vi "ITX to LV 2.2.vi"(0 "file (use dialog)":path=path "P:/sample/GaAs/GaAs quantum dots/2008/PL Map/A1 735/060731ASBA_A1_6.0.itx") -> (2 "2D array":dbl[][](array[numeric]), 3 "1D arrays":dbl[][](array[numeric]), 4 "wave names":string[](array[string]), 5 "Notes":string)   [LabVIEW 2016, in "LVtoITX.lvclass"]
uses:
  LVtoITX.lvclass
panel:
  out "variant to data (ms)":u32
  out "Commands":string
  out "parse 2 (ms)":u32
  out "text to data (ms)":u32
  out "parse 1 (ms)":u32
  out "open file (ms)":u32
  out "Array 4":i32[](array[numeric])
  out "Array":string[](array[string])
  out "array":string[](array[string])
  out "error out":errorcluster
  out "logical AND":bool
  out "Array 2":string[](array[string])
  out "spreadsheet strings":string[](array[string])
  in  "error in":errorcluster
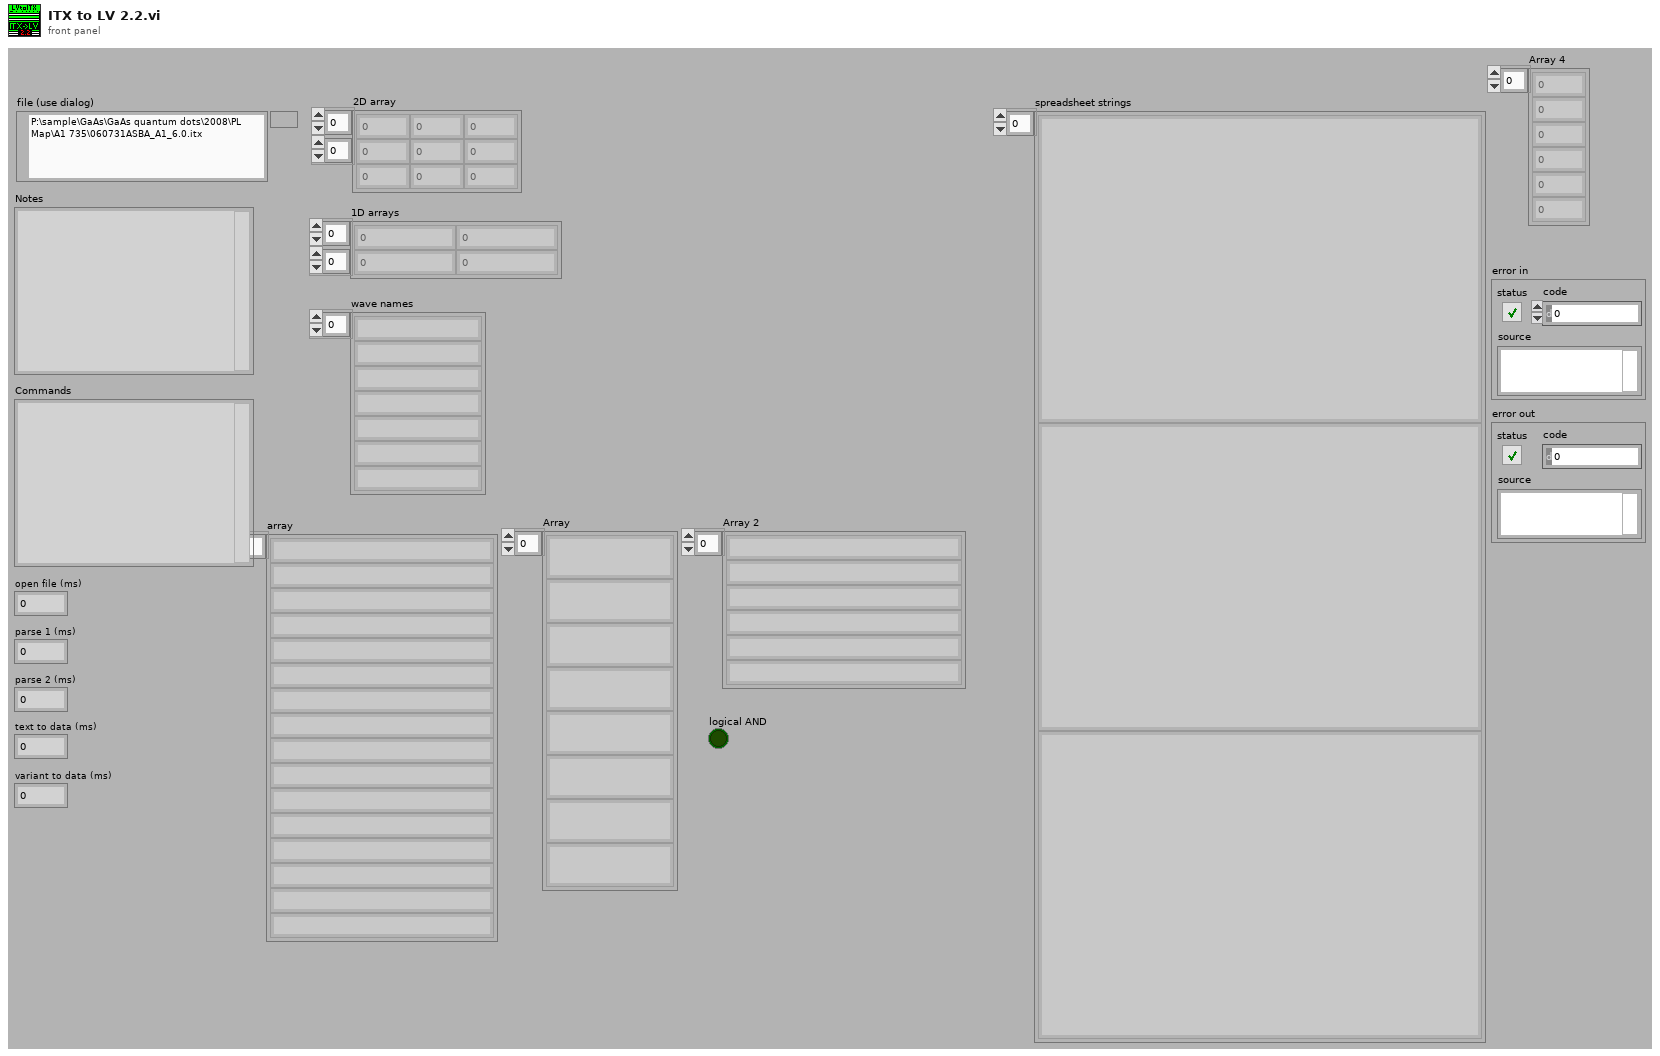
[diagram p1: front panel]
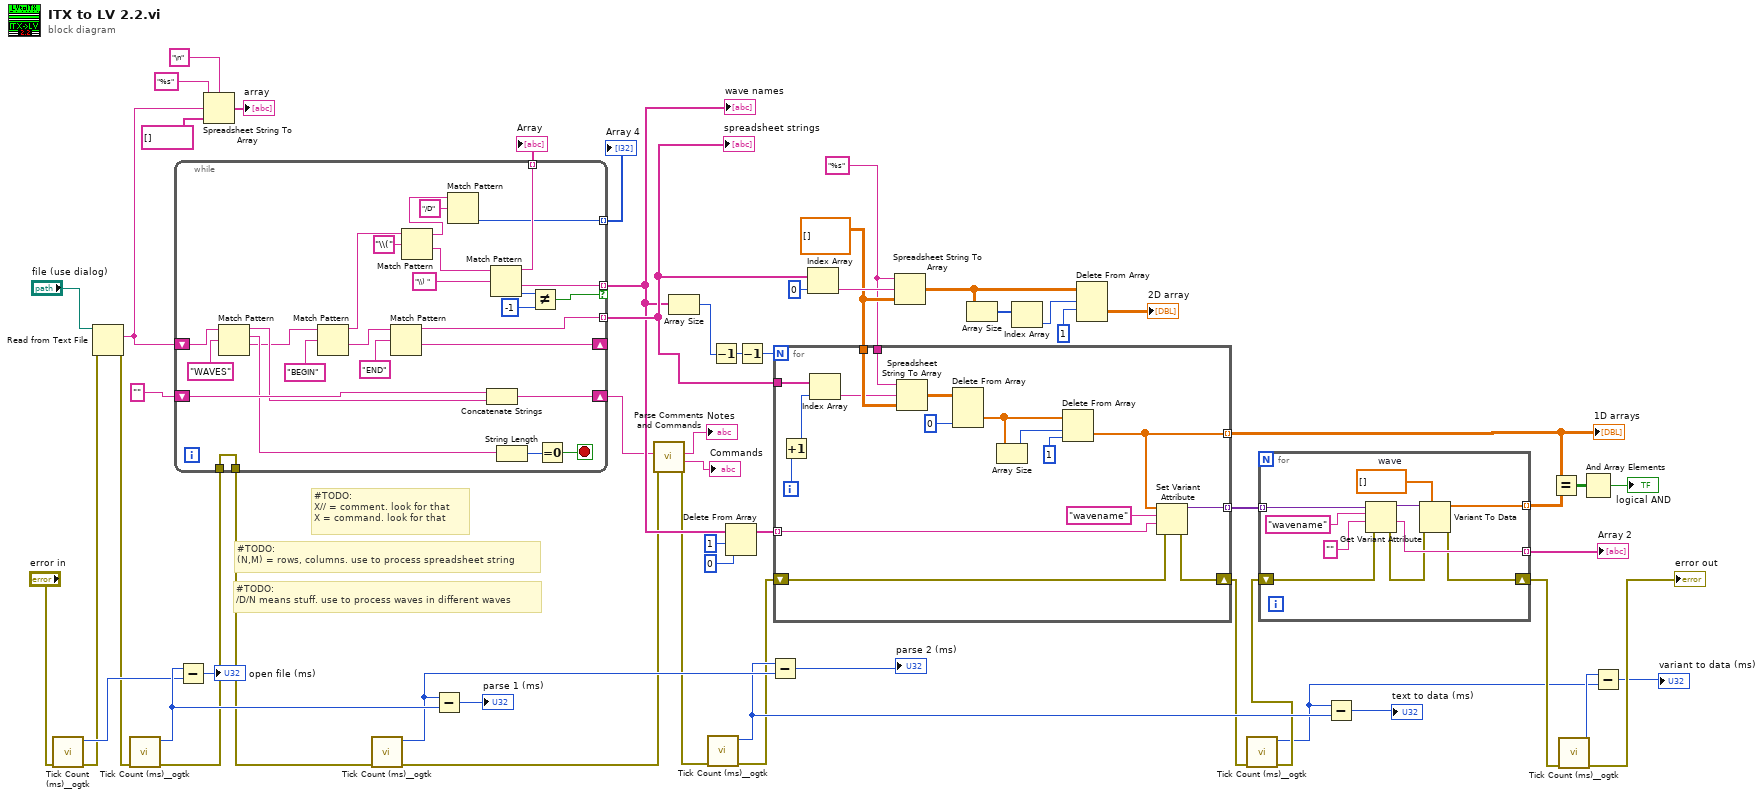
[diagram p0: block diagram]
diagram:
  w50 = "%s" ("format string")
  w51 = dbl[][] [] ("array type (2D Dbl)")
  # "#TODO:\n/D/N means stuff. use to process waves in different waves"
  # "#TODO:\n(N,M) = rows, columns. use to process spreadsheet string"
  # "#TODO:\nX// = comment. look for that\nX = command. look for that"
  n1 = call <userlib>:"Tick Count (ms)__ogtk.vi"("error in (no error)"="error in") -> ("error out"=w17:errorcluster, "millisecond timer value"=w20:u32)  [unwired: 9 in]
  n2 = Read from Text File(file (use dialog)="file (use dialog)", error in=w17) -> (text=w30:string, error out=w9:errorcluster)  [unwired: 1 in, 3 out]
  n3 = call <userlib>:"Tick Count (ms)__ogtk.vi"("error in (no error)"=w9) -> ("error out"=w16:errorcluster, "millisecond timer value"=w24:u32)  [unwired: 9 in]
  n4 = while {
    tunnel: [w64] -> w35 mode=indexing
    shift-right: [w84] -> _
    shift-left: w30 -> [w76]
    tunnel: [w68] -> w34 mode=indexing if=w60
    shift-right: [w78] -> w14
    shift-left: "" ("regular expression") -> [w77]
    tunnel: [w70] -> w28 mode=indexing
    tunnel: [w65] -> w27 mode=indexing
    tunnel: w16 -> [w59]
    tunnel: [w59] -> w15
    stop <- w63 stop-if-true
    n5 = Match Pattern(string=w76, regular expression="WAVES") -> (before substring=w74:string, match substring=w75:string, after substring=w73:string)  [unwired: 2 out]
    n6 = Match Pattern(string=w73, regular expression="BEGIN" ("regular expression 2")) -> (before substring=w71:string, after substring=w85:string)  [unwired: 3 out]
    n7 = Match Pattern(string=w85, regular expression="END" ("regular expression 3")) -> (before substring=w64:string, after substring=w84:string)  [unwired: 3 out]
    n8 = Match Pattern(string=w71, regular expression="\\(") -> (before substring=w66:string, after substring=w69:string)  [unwired: 3 out]
    n9 = Match Pattern(string=w66, regular expression="/D") -> (offset past match=w65:i32)  [unwired: 4 out]
    n10 = Concatenate Strings(w77, w74) -> (w78:string)
    n11 = Match Pattern(string=w69, regular expression="\\) ") -> (before substring=w70:string, after substring=w68:string, offset past match=w62:i32)  [unwired: 2 out]
    n12 = String Length(string=w75) -> (length=w83:i32)
    n13 = Not Equal?(x=w62, y=-1) -> (x != y?=w60:bool)
    n14 = Equal To 0?(x=w83) -> (x = 0?=w63:bool)
  }
  "wave names" <- w34
  "spreadsheet strings" <- w35
  "Array" <- w28
  "Array 4" <- w27
  n15 = Subtract(x=w24, y=w20) -> (x-y=→"open file (ms)":u32)
  n16 = Spreadsheet String To Array(delimiter (Tab)="\n", format string="%s", spreadsheet string=w30, array type (2D Dbl)=string[] []) -> (array=→"array":string[])
  n17 = call <userlib>:"Tick Count (ms)__ogtk.vi"("error in (no error)"=w15) -> ("error out"=w11:errorcluster, "millisecond timer value"=w22:u32)  [unwired: 9 in]
  n18 = Subtract(x=w22, y=w24) -> (x-y=→"parse 1 (ms)":u32)
  n19 = call "Parse Comments and Commands.vi"("error in"=w11, "Igor Comments and Commands"=w14) -> ("error out"=w10:errorcluster, "Commands"=→"Commands":string, "Comments"=→"Notes":string)  [unwired: 7 in]
  n20 = Array Size(array=w34) -> (size(s)=w36:i32)
  n21 = call <userlib>:"Tick Count (ms)__ogtk.vi"("error in (no error)"=w10) -> ("error out"=w8:errorcluster, "millisecond timer value"=w19:u32)  [unwired: 9 in]
  n22 = Decrement(x=w36) -> (x-1=w49:i32)
  n23 = Delete From Array(array=w34, length=1, index=0) -> (array with subset deleted=w44:string[])  [unwired: 1 out]
  n24 = Decrement(x=w49) -> (x-1=w48:i32)
  n25 = Subtract(x=w19, y=w22) -> (x-y=→"parse 2 (ms)":u32)
  n26 = for {
    N: w48 -> [_]
    tunnel: [w86] -> w39 mode=indexing
    tunnel: w51 -> [w97]
    tunnel: w35 -> [w96]
    tunnel: w50 -> [w95]
    tunnel: w44 -> [w90] mode=indexing
    tunnel: [w89] -> w41 mode=indexing
    shift-right: [w88] -> w7
    shift-left: w8 -> [w87]
    i -> [w94]
    n27 = Increment(x=w94) -> (x+1=w93:i32)
    n28 = Index Array(array=w96, index=w93) -> (element=w92:string)
    n29 = Spreadsheet String To Array(format string=w95, spreadsheet string=w92, array type (2D Dbl)=w97) -> (array=w101:dbl[][])  [unwired: 1 out]
    n30 = Delete From Array(array=w101, index (col)=0 ("disabled index (col)")) -> (deleted portion=w100:dbl[])  [unwired: 2 in, 1 out]
    n31 = Array Size(array=w100) -> (size(s)=w99:i32)
    n32 = Delete From Array(array=w100, length=w99, index=1) -> (deleted portion=w86:dbl[])  [unwired: 1 out]
    n33 = Set Variant Attribute(Variant=w86, name="wavename", value=w90, error in=w87) -> (Variant out=w89:variant, error out=w88:errorcluster)  [unwired: 1 out]
  }
  "1D arrays" <- w39
  n34 = Index Array(array=w35, index=0) -> (element=w57:string)
  n35 = Spreadsheet String To Array(format string=w50, spreadsheet string=w57, array type (2D Dbl)=w51) -> (array=w55:dbl[][])  [unwired: 1 out]
  n36 = Array Size(array=w55) -> (size(s)=w54:i32[])
  n37 = Index Array(array=w54) -> (element=w52:i32)  [unwired: 1 in]
  n38 = Delete From Array(array=w55, length=w52, index (row)=1) -> (deleted portion=→"2D array":dbl[][])  [unwired: 1 in, 1 out]
  n39 = call <userlib>:"Tick Count (ms)__ogtk.vi"("error in (no error)"=w7) -> ("error out"=w6:errorcluster, "millisecond timer value"=w1:u32)  [unwired: 9 in]
  n40 = for {
    tunnel: [w109] -> w42 mode=indexing
    tunnel: w41 -> [w110] mode=indexing
    shift-right: [w104] -> w5
    shift-left: w6 -> [w103]
    tunnel: [w105] -> w40 mode=indexing
    w106 = dbl[] []  # wave
    n41 = Get Variant Attribute(Variant=w110, name="wavename", default value (empty Variant)="" ("name"), error in=w103) -> (duplicate Variant=w107:variant, value=w109:string, error out=w108:errorcluster)  [unwired: 1 out]
    n42 = Variant To Data(error in=w108, type=w106, Variant=w107) -> (data=w105:dbl[], error out=w104:errorcluster)
  }
  "Array 2" <- w42
  n43 = Subtract(x=w1, y=w19) -> (x-y=→"text to data (ms)":u32)
  n44 = Equal?(x=w39, y=w40) -> (x = y?=w38:bool[][])
  n45 = call <userlib>:"Tick Count (ms)__ogtk.vi"("error in (no error)"=w5) -> ("error out"=→"error out":errorcluster, "millisecond timer value"=w2:u32)  [unwired: 9 in]
  n46 = And Array Elements(Boolean array=w38) -> (logical AND=→"logical AND":bool)
  n47 = Subtract(x=w2, y=w1) -> (x-y=→"variant to data (ms)":u32)
